vi "filter pipe - plot staff.vi"(0 "omega  in":dbl[](array[numeric]), 1 "zin":cdb[](array[numeric]), 2 "z out":cdb[](array[numeric]), 4 "smart filter: span":dbl(slide)=0.1 min=0.0001 max=0.5 step=0.001 scale=0.001..0.5 scale format="%#_2g", 5 "tale of three indices -- int -- control":T1={"left"=0, "center"=0, "right"=0, "right most"=0, "left most"=0, "window"=0, "max win factor"=2, "max win"=2, "min win"=2}, 6 "center":cdb, 7 "Plot: complex plane - filter":refnum<vi>, 8 "norm":dbl, 9 "Plot: fragment":refnum<vi>) -> ()   [LabVIEW 2012]
uses:
  tale of three indices -- int -- control.ctl
  generate linear region.vi
panel:
  out "size(s) 2":i32
  out "size(s)":i32
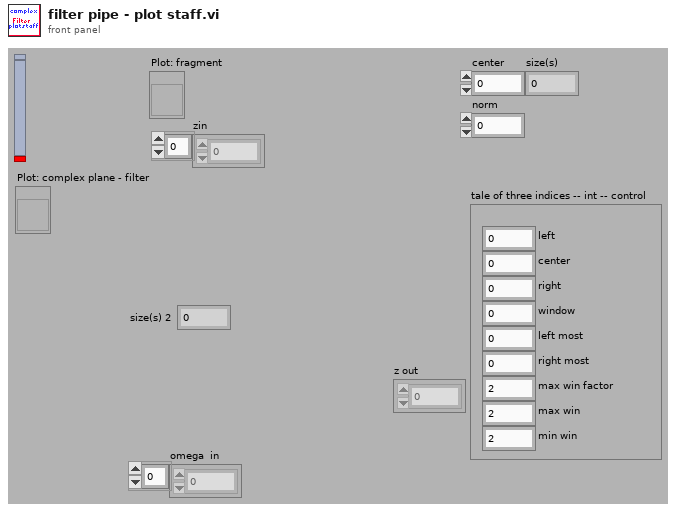
[diagram p1: front panel]
types:
  T1 = typedef "tale of three indices -- int -- control.ctl" = cluster{"left":i32, "center":i32, "right":i32, "right most":i32, "left most":i32, "window":i32, "max win factor":i32, "max win":i32, "min win":i32}
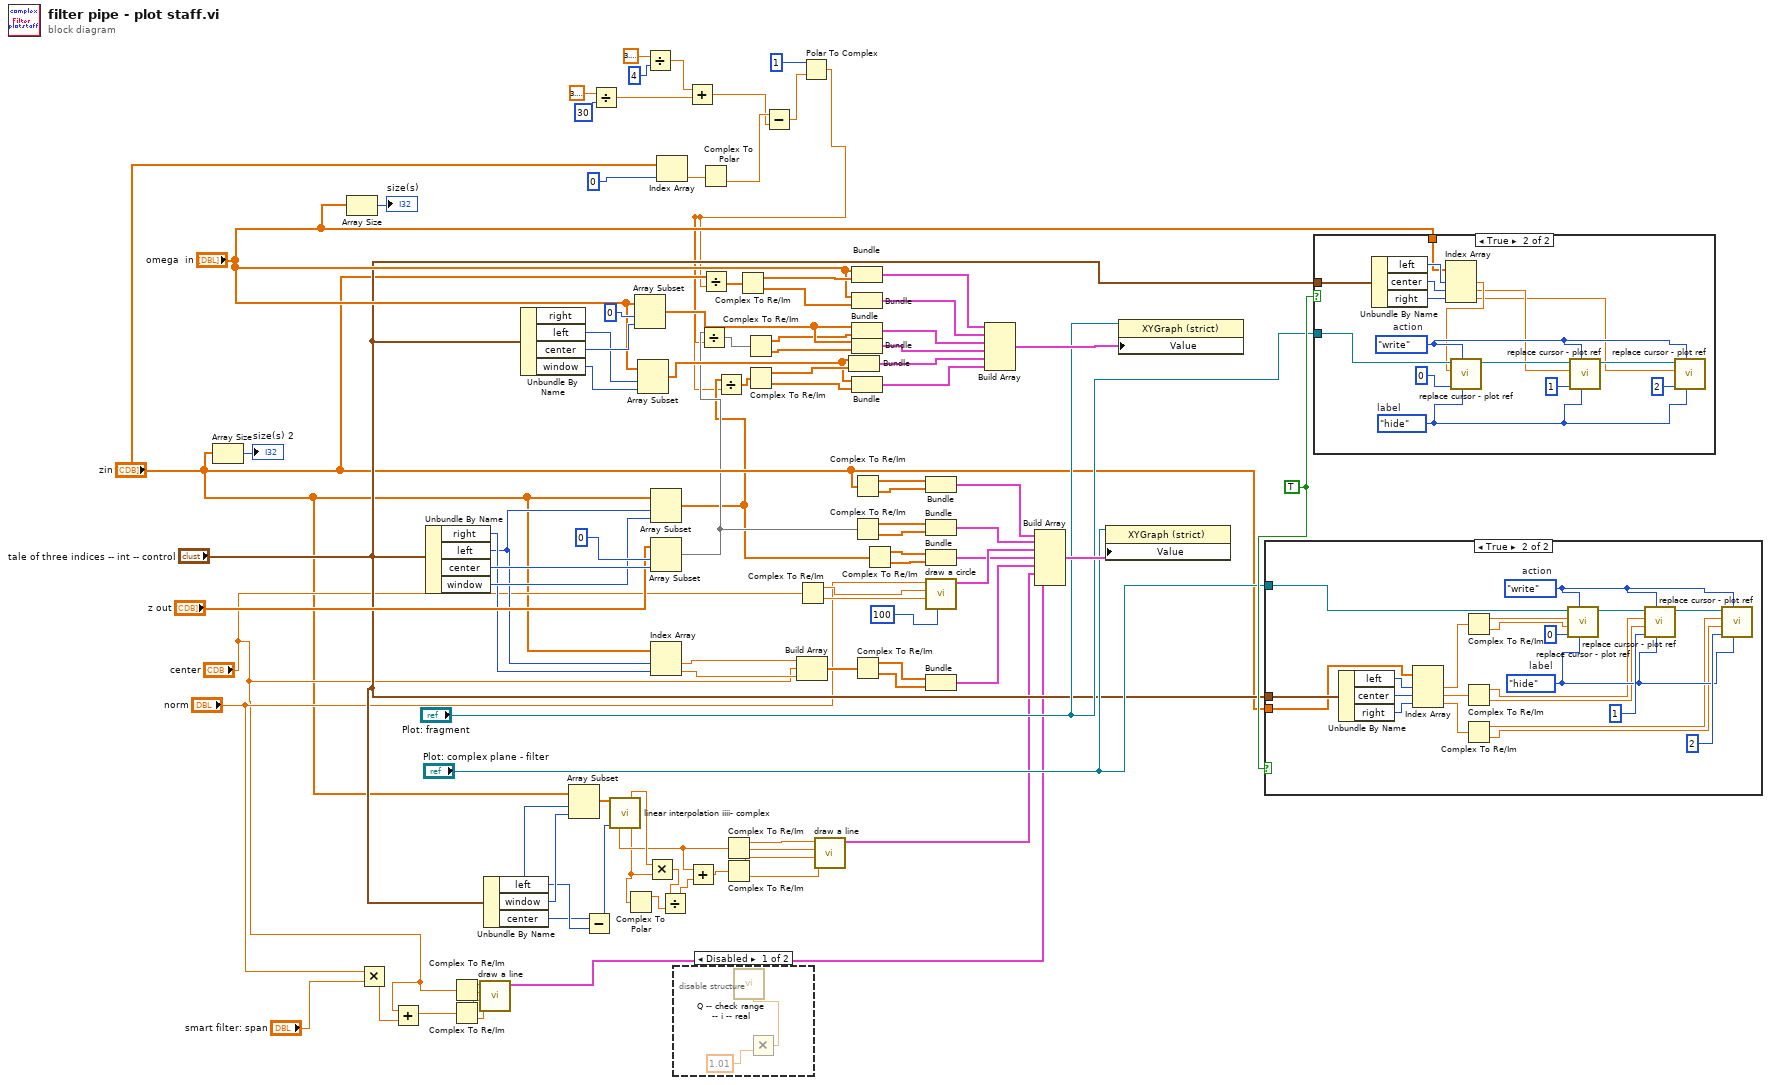
[diagram p0: block diagram]
diagram:
  w71 = TRUE
  n1 = Array Size(array="zin") -> (size(s)=→"size(s) 2":i32)
  n2 = Array Size(array="omega  in") -> (size(s)=→"size(s)":i32)
  n3 = Multiply(x="norm", y="smart filter: span") -> (x*y=w22:dbl)
  n4 = Add(x="center", y=w22) -> (x+y=w21:cdb)
  n5 = Unbundle By Name("tale of three indices -- int -- control") -> ("right"=w53:i32, "left"=w48:i32, "center"=w58:i32, "window"=w54:i32)
  n6 = Complex To Re/Im(x + iy="center") -> (x=w27:dbl, y=w24:dbl)
  n7 = Complex To Re/Im(x + iy=w21) -> (x=w25:dbl, y=w26:dbl)
  n8 = call "draw a line.vi"("y1"=w26, "y0"=w24, "x1"=w25, "x0"=w27) -> ("output cluster"=w20:cluster{dbl[], dbl[]})  [unwired: 7 in]
  n9 = Unbundle By Name("tale of three indices -- int -- control") -> ("left"=w45:i32, "window"=w46:i32, "center"=w44:i32)
  n10 = Unbundle By Name("tale of three indices -- int -- control") -> ("left"=w73:i32, "center"=w75:i32, "window"=w72:i32)  [unwired: 1 out]
  n11 = Array Subset(array="zin", index=w45, length=w46) -> (w47:cdb[])
  n12 = Subtract(x=w44, y=w45) -> (x-y=w43:i32)
  n13 = Divide(x=3.141592653589793, y=30) -> (x/y=w1:dbl)
  n14 = call "linear interpolation iiii- complex.vi"("Array"=w47, "center"=w43) -> ("directed sigma"=w40:dbl, "intercept"=w39:cdb, "slope"=w33:cdb)  [unwired: 5 in, 6 out]
  n15 = Complex To Polar(r * e^(i*theta)=w33) -> (r=w32:dbl)  [unwired: 1 out]
  n16 = Array Subset(array="omega  in", index=0, length=w75) -> (w74:dbl[])
  n17 = Array Subset(array="omega  in", index=w73, length=w72) -> (w62:dbl[])
  n18 = Divide(x=3.141592653589793, y=4) -> (x/y=w5:dbl)
  n19 = Multiply(x=w40, y=w33) -> (x*y=w31:cdb)
  n20 = Array Subset(array="zin", index=w48, length=w54) -> (w13:cdb[])
  n21 = Array Subset(array="z out", index=0, length=w58) -> (w15:cdb[])
  n22 = Index Array(array="zin", index #1=w48, index #2=w53) -> (element #1=w56:cdb, element #2=w55:cdb)
  n23 = Index Array(array="zin", index=0) -> (element=w17:cdb)
  n24 = Divide(x=w31, y=w32) -> (x/y=w30:cdb)
  n25 = disable-structure shown="Disabled" {
    frame Disabled {
      n26 = Multiply(y=1.01) -> (x*y=w99:dbl)  [unwired: 1 in]
      n27 = call "Q -- check range -- i -- real.vi"("upper"=w99) -> ()  [unwired: 8 in, 3 out]
    }
    frame Enabled {
    }
  }
  n28 = Add(x=w5, y=w1) -> (x+y=w4:dbl)
  n29 = Add(x=w39, y=w30) -> (x+y=w38:cdb)
  n30 = Complex To Polar(r * e^(i*theta)=w17) -> (theta=w8:dbl)  [unwired: 1 out]
  n31 = Complex To Re/Im(x + iy=w39) -> (x=w41:dbl, y=w34:dbl)
  n32 = Complex To Re/Im(x + iy=w38) -> (x=w35:dbl, y=w37:dbl)
  n33 = Subtract(x=w8, y=w4) -> (x-y=w7:dbl)
  n34 = Build Array(w56, "center", w55) -> (w52:cdb[])
  n35 = Complex To Re/Im(x + iy="center") -> (x=w92:dbl, y=w91:dbl)
  n36 = Polar To Complex(1:w7, 2:1) -> (0:w6:cdb)
  n37 = Divide(x=w15, y=w6) -> (x/y=w14:cdb[])
  n38 = Divide(x="zin", y=w6) -> (x/y=w16:cdb[])
  n39 = Divide(x=w13, y=w6) -> (x/y=w12:cdb[])
  n40 = Complex To Re/Im(x + iy=w16) -> (x=w79:dbl[], y=w78:dbl[])
  n41 = Complex To Re/Im(x + iy=w14) -> (x=w68:dbl[], y=w67:dbl[])
  n42 = Complex To Re/Im(x + iy=w12) -> (x=w64:dbl[], y=w63:dbl[])
  n43 = call "draw a line.vi"("y1"=w37, "y0"=w34, "x1"=w35, "x0"=w41) -> ("output cluster"=w36:cluster{dbl[], dbl[]})  [unwired: 7 in]
  n44 = Bundle(w62, w64) -> (w61:cluster{dbl[], dbl[]})  [unwired: 1 in]
  n45 = Bundle("omega  in"="omega  in", w79) -> (w77:cluster{"omega  in":dbl[], dbl[]})  [unwired: 1 in]
  n46 = Bundle("omega  in"="omega  in", w78) -> (w81:cluster{"omega  in":dbl[], dbl[]})  [unwired: 1 in]
  n47 = Bundle(w74, w68) -> (w66:cluster{dbl[], dbl[]})  [unwired: 1 in]
  n48 = Bundle(w74, w67) -> (w65:cluster{dbl[], dbl[]})  [unwired: 1 in]
  n49 = Bundle(w62, w63) -> (w60:cluster{dbl[], dbl[]})  [unwired: 1 in]
  n50 = Complex To Re/Im(x + iy="zin") -> (x=w98:dbl[], y=w97:dbl[])
  n51 = Complex To Re/Im(x + iy=w15) -> (x=w96:dbl[], y=w95:dbl[])
  n52 = Complex To Re/Im(x + iy=w52) -> (x=w84:dbl[], y=w83:dbl[])
  n53 = Complex To Re/Im(x + iy=w13) -> (x=w87:dbl[], y=w86:dbl[])
  n54 = Bundle(w98, w97) -> (w94:cluster{dbl[], dbl[]})  [unwired: 1 in]
  n55 = Bundle(w96, w95) -> (w93:cluster{dbl[], dbl[]})  [unwired: 1 in]
  n56 = Bundle(w87, w86) -> (w85:cluster{dbl[], dbl[]})  [unwired: 1 in]
  n57 = call "draw a circle.vi"("number of points"=100, "center Y"=w91, "center x"=w92, "radius"="norm") -> ("output cluster"=w89:cluster{dbl[], dbl[]})  [unwired: 7 in]
  n58 = Bundle(w84, w83) -> (w82:cluster{dbl[], dbl[]})  [unwired: 1 in]
  n59 = Build Array(w77, w81, w66, w65, w61, w60) -> (w80:cluster{"omega  in":dbl[], dbl[]}[])
  n60 = Build Array(w94, w93, w89, w85, w82, w36, w20) -> (w88:cluster{dbl[], dbl[]}[])
  n61 = property class="XYGraph (strict)"(reference="Plot: complex plane - filter", "Value"=w88) -> ()  [unwired: 1 in, 2 out]
  n62 = property class="XYGraph (strict)"(reference="Plot: fragment", "Value"=w80) -> ()  [unwired: 1 in, 2 out]
  n63 = case shown="True" w71 {
    tunnel: "tale of three indices -- int -- control" -> [_ w115]
    tunnel: "zin" -> [_ w114]
    tunnel: "Plot: complex plane - filter" -> [_ w113]
    frame False {
    }
    frame True {
      w116 = enum16{"hide", "show x", "show y", "show (x,y)"}."hide"  # label
      w122 = enum16{"", "read", "write"}."write"  # action
      n64 = Unbundle By Name(w115) -> ("left"=w112:i32, "center"=w111:i32, "right"=w110:i32)
      n65 = Index Array(array=w114, index #1=w112, index #2=w111, index #3=w110) -> (element #1=w107:cdb, element #2=w108:cdb, element #3=w109:cdb)
      n66 = Complex To Re/Im(x + iy=w107) -> (x=w106:dbl, y=w105:dbl)
      n67 = Complex To Re/Im(x + iy=w108) -> (x=w104:dbl, y=w103:dbl)
      n68 = Complex To Re/Im(x + iy=w109) -> (x=w102:dbl, y=w101:dbl)
      n69 = call "replace cursor - plot ref.vi"("label"=w116, "action"=w122, "cursor index"=0, "new  Y"=w105, "new X"=w106, "Plot ref in"=w113) -> ("Plot ref out"=w118:refnum<vi>)  [unwired: 3 in, 2 out]
      n70 = call "replace cursor - plot ref.vi"("label"=w116, "action"=w122, "cursor index"=1, "new  Y"=w103, "new X"=w104, "Plot ref in"=w118) -> ("Plot ref out"=w117:refnum<vi>)  [unwired: 3 in, 2 out]
      n71 = call "replace cursor - plot ref.vi"("label"=w116, "action"=w122, "cursor index"=2, "new  Y"=w101, "new X"=w102, "Plot ref in"=w117) -> ()  [unwired: 3 in, 3 out]
    }
  }
  n72 = case shown="True" w71 {
    tunnel: "tale of three indices -- int -- control" -> [_ w131]
    tunnel: "Plot: fragment" -> [_ w127]
    tunnel: "omega  in" -> [_ w126]
    frame False {
    }
    frame True {
      w132 = enum16{"hide", "show x", "show y", "show (x,y)"}."hide"  # label
      w138 = enum16{"", "read", "write"}."write"  # action
      n73 = Unbundle By Name(w131) -> ("left"=w130:i32, "center"=w129:i32, "right"=w128:i32)
      n74 = Index Array(array=w126, index #1=w130, index #2=w129, index #3=w128) -> (element #1=w125:dbl, element #2=w124:dbl, element #3=w123:dbl)
      n75 = call "replace cursor - plot ref.vi"("label"=w132, "action"=w138, "cursor index"=0, "new X"=w125, "Plot ref in"=w127) -> ("Plot ref out"=w134:refnum<vi>)  [unwired: 4 in, 2 out]
      n76 = call "replace cursor - plot ref.vi"("label"=w132, "action"=w138, "cursor index"=1, "new X"=w124, "Plot ref in"=w134) -> ("Plot ref out"=w133:refnum<vi>)  [unwired: 4 in, 2 out]
      n77 = call "replace cursor - plot ref.vi"("label"=w132, "action"=w138, "cursor index"=2, "new X"=w123, "Plot ref in"=w133) -> ()  [unwired: 4 in, 3 out]
    }
  }
